vi "r_dual.vi"(1 "object cluster":T1, 2 "constraints cluster":T2, 3 "lmd_input":dbl[](array[numeric]), 4 "q_input":dbl[](array[numeric])) -> (0 "dual residual":dbl[](array[numeric]))   [LabVIEW 2019]
panel:
  # "input : constraints cluster\n            object cluster\n            q_input\n            lmd_input"
  # "output : dual residual, \n               matrix, n*1"
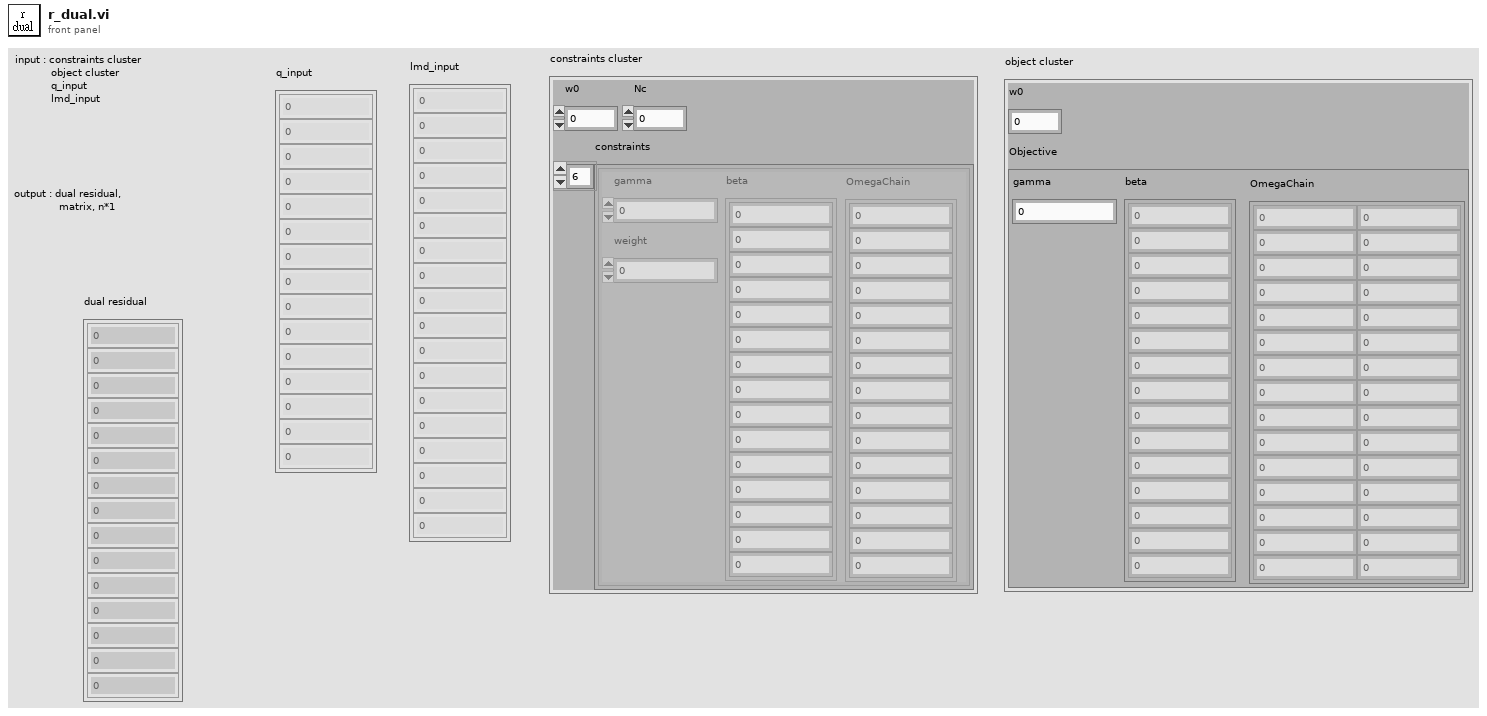
[diagram p1: front panel]
types:
  T1 = cluster{"w0":dbl, "Objective":cluster{"beta":dbl[], "gamma":dbl, "OmegaChain":dbl[][]}}
  T2 = cluster{"w0":dbl, "constraints":cluster{"beta":dbl[], "gamma":dbl, "OmegaChain":dbl[], "weight":dbl}[], "Nc":i32}
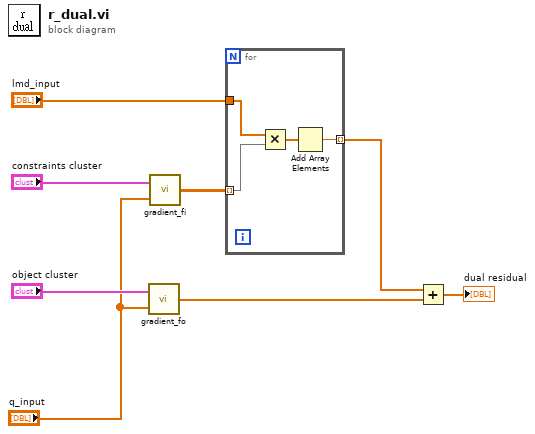
[diagram p0: block diagram]
diagram:
  n1 = call "gradient_fo.vi"("q_input"="q_input", "Object cluster"="object cluster") -> ("Gradient of fo"=w3:dbl[])
  n2 = call "gradient_fi.vi"("q_input"="q_input", "constraints cluster"="constraints cluster") -> ("gradient of fi"=w5:dbl[][])
  n3 = for {
    tunnel: w5 -> [w12] mode=indexing
    tunnel: "lmd_input" -> [w11]
    tunnel: [w9] -> w2 mode=indexing
    n4 = Multiply(x=w11, y=w12) -> (x*y=w10:dbl[])
    n5 = Add Array Elements(numeric array=w10) -> (sum=w9:dbl)
  }
  n6 = Add(x=w2, y=w3) -> (x+y=→"dual residual":dbl[])
